vi "Autonomous.vi"(11 "Call Context":T8) -> (0 "SubState 2":T1, 1 "Loop 2 Data":T4, 2 "SubState 1":T1, 3 "Loop 1 Data":T5, 4 "Loop 3 Data":T3, 5 "SubState 0":T1=enum."driver control", 6 "SubState 3":T1, 7 "Loop 0 Data":T6, 8 "SubState 4":T1, 9 "Loop 4 Data":T2, 10 "SubState 5":T7)   [LabVIEW 2013]
uses:
  typedefs/state machine/subStates.ctl
  <vilib>/Rock Robotics/WPI/DriverStation/WPI_DriverStationDerivedRobotMode.ctl
  typedefs/state machine/singleUseSubstate.ctl
  typedefs/loop datatypes/Loop 0 Datatype.ctl
  typedefs/loop datatypes/Loop 1 Datatype.ctl
  typedefs/loop datatypes/Loop 2 Datatype.ctl
  typedefs/loop datatypes/Loop 3 Datatype.ctl
  typedefs/loop datatypes/Loop 4 Datatype.ctl
  typedefs/fg_getset.ctl
  typedefs/vision/vision enable.ctl
panel:
  # "Autonomous Loop Data and Substates"
  # "Robot Drive"
  # "Loop 1"
  # "Loop 2"
  # "Loop 3"
  # "Loop 4"
  # "Pneumatics"
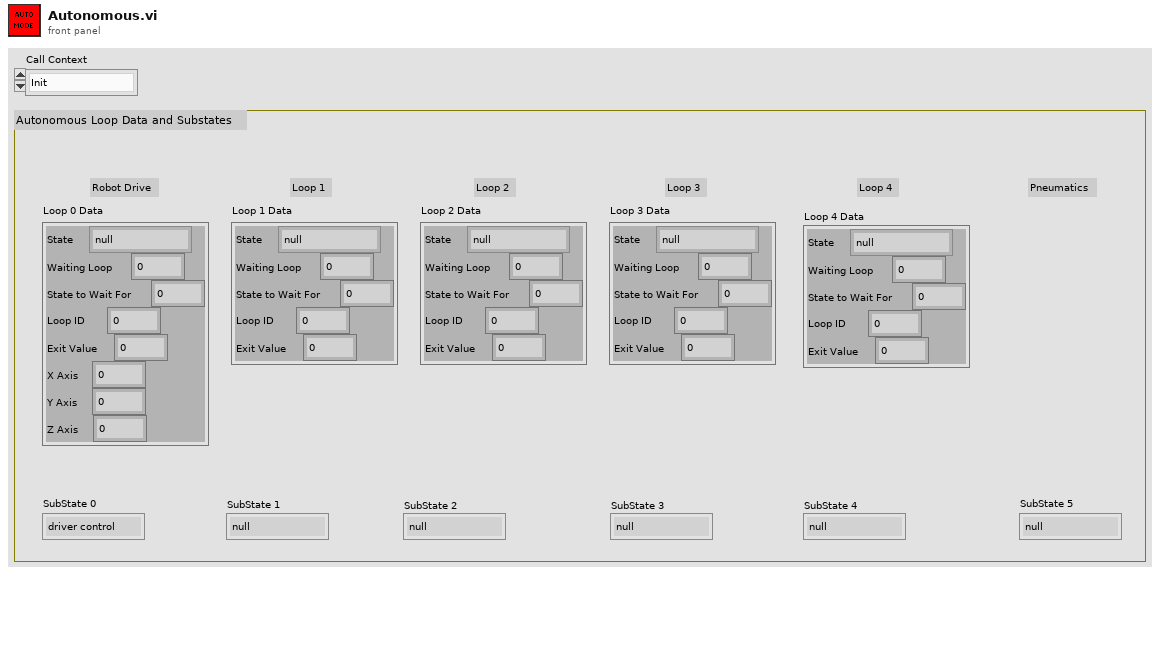
[diagram p1: front panel]
types:
  T1 = typedef "subStates.ctl" = enum16{"null", "wait", "driver control", "auto", "manual override", "hold position", "rotate", "test", "end"}
  T2 = typedef "Loop 4 Datatype.ctl" = cluster{"State":T1, "Waiting Loop":i32, "State to Wait For":i32, "Loop ID":i32, "Exit Value":i32}
  T3 = typedef "Loop 3 Datatype.ctl" = cluster{"State":T1, "Waiting Loop":i32, "State to Wait For":i32, "Loop ID":i32, "Exit Value":i32}
  T4 = typedef "Loop 2 Datatype.ctl" = cluster{"State":T1, "Waiting Loop":i32, "State to Wait For":i32, "Loop ID":i32, "Exit Value":i32}
  T5 = typedef "Loop 1 Datatype.ctl" = cluster{"State":T1, "Waiting Loop":i32, "State to Wait For":i32, "Loop ID":i32, "Exit Value":i32}
  T6 = typedef "Loop 0 Datatype.ctl" = cluster{"State":T1, "Waiting Loop":i32, "State to Wait For":i32, "Loop ID":i32, "Exit Value":i32, "X Axis":dbl, "Y Axis":dbl, "Z Axis":dbl}
  T7 = typedef "singleUseSubstate.ctl" = enum16{"null", "wait", "shift high", "shift low", "end"}
  T8 = typedef "WPI_DriverStationDerivedRobotMode.ctl" = enum16{"Init", "Execute", "Stop"}
  T9 = typedef "vision enable.ctl" = enum16{"Enable", "Disable", "Stop"}
  T10 = typedef "fg_getset.ctl" = enum16{"Get", "Set"}
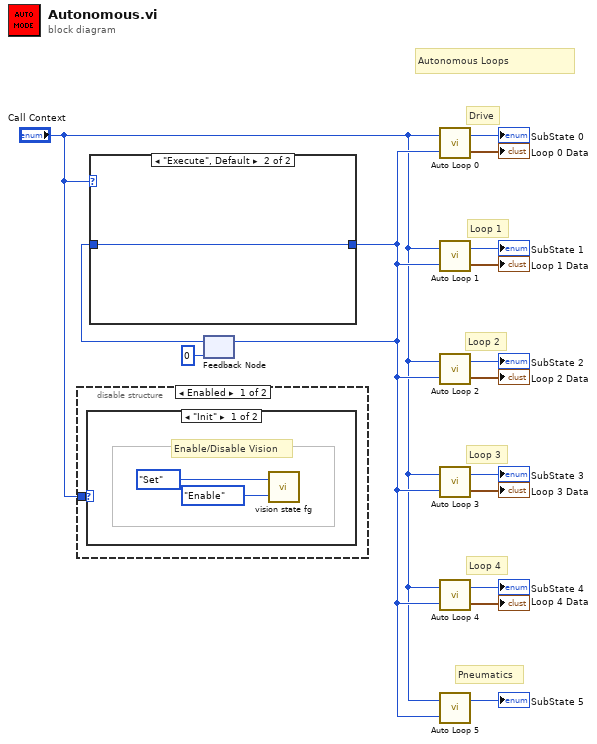
[diagram p0: block diagram]
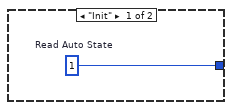
[diagram p4: hidden frame]
diagram:
  # "Loop 4"
  # "Autonomous Loops"
  # "Loop 3"
  # "Loop 2"
  # "Pneumatics"
  # "Loop 1"
  # "Drive"
  n1 = disable-structure shown="Enabled" {
    disable-tunnel: "Call Context" -> [w16 _]
    frame Enabled {
      n2 = case shown="\"Init\"" w16 {
        frame "Init" {
          # "Enable/Disable Vision"
          n3 = call "vision state fg.vi"("Action"=vision_enable."Enable", "Menu"=fg_getset."Set") -> ()  [unwired: 2 out]
        }
        frame "Execute", Default {
        }
      }
    }
    frame Disabled {
    }
  }
  n4 = feedback #1(u8 0 ("Read Auto State")) -> (w4:u8)
  n5 = case shown="\"Execute\", Default" "Call Context" {
    tunnel: [w19 w20] -> w15
    tunnel: w4 -> [_ w20]
    frame "Init" {
      w19 = u8 1  # Read Auto State
    }
    frame "Execute", Default {
    }
  }
  n6 = feedback-in #1(w15) -> ()
  n7 = call "Auto Loop 0.vi"("Auto State"=w15, "Call Context"="Call Context") -> ("Loop 0 Data"=→"Loop 0 Data":T6, "SubState 0"=→"SubState 0":T1)
  n8 = call "Auto Loop 1.vi"("Auto State"=w15, "Call Context"="Call Context") -> ("Loop 1 Data"=→"Loop 1 Data":T5, "SubState 1"=→"SubState 1":T1)
  n9 = call "Auto Loop 2.vi"("Auto State"=w15, "Call Context"="Call Context") -> ("Loop 2 Data"=→"Loop 2 Data":T4, "SubState 2"=→"SubState 2":T1)
  n10 = call "Auto Loop 3.vi"("Auto State"=w15, "Call Context"="Call Context") -> ("Loop 3 Data"=→"Loop 3 Data":T3, "SubState 3"=→"SubState 3":T1)
  n11 = call "Auto Loop 4.vi"("Auto State"=w15, "Call Context"="Call Context") -> ("Loop 4 Data"=→"Loop 4 Data":T2, "SubState 3"=→"SubState 4":T1)
  n12 = call "Auto Loop 5.vi"("Auto State"=w15, "Call Context"="Call Context") -> ("SubState 5"=→"SubState 5":T7)  [unwired: 1 in]
